vi "wait_init_01.vi"   [LabVIEW 2011]
uses:
  wait_globals.vi
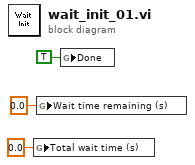
[diagram p0: block diagram]
diagram:
  n1 = global write "wait_globals.vi" "Total wait time (s)"(0.0 ("Total wait time (s)")) -> ()
  n2 = global write "wait_globals.vi" "Wait time remaining (s)"(0.0 ("Wait time remaining (s)")) -> ()
  n3 = global write "wait_globals.vi" "Done"(TRUE ("Done")) -> ()
